vi "principal.vi"() -> ()   [LabVIEW 2020]
uses:
  <vilib>/Utility/file.llb/Read Delimited Spreadsheet (string).vi
  <vilib>/Utility/file.llb/Write Delimited Spreadsheet (string).vi
panel:
  in  "stop 2":bool
  in  "file path (dialog if empty) 2":path
  in  "stop":bool
  in  "file path (dialog if empty)":path
  out "appended path":path
  in  "CONTROL B":T1(tab)
  in  "Usuario 2":string
  in  "ingresar 2":bool
  in  "Contraseña 2":string
  out "String 4":string
  in  "volver 5":bool
  in  "Eliminar  2":bool
  in  "Agregar  2":bool
  in  "volver 6":bool
  in  "Agregar  10":bool
  in  "Contraseña nueva 2":string
  in  "Usuario nuevo 2":string
  out "String 3":string
  in  "volver 7":bool
  in  "Fila a eliminar 2":i32
  in  "Eliminar  4":bool
  out "all rows 2":string[][](array[string])
  in  "volver 10":bool
  out "Hora del sistema 2":string
  in  "volver 8":bool
  out "Nombre del usuario 2":string
  in  "CONTROL A":T2(tab)
  in  "ingresar":bool
  in  "Contraseña":string
  in  "Usuario":string
  in  "Agregar  3":bool
  in  "volver":bool
  in  "Eliminar":bool
  in  "Contraseña nueva":string
  in  "Usuario nuevo":string
  in  "volver 3":bool
  in  "Agregar":bool
  out "String":string
  in  "volver 4":bool
  out "all rows":string[][](array[string])
  in  "Fila a eliminar":i32
  in  "Eliminar  3":bool
  in  "volver 9":bool
  out "Hora del sistema":string
  out "Nombre del usuario":string
  in  "volver 2":bool
  # "INGRESAR"
  # "ADMINISTRADOR"
  # "PRINCIPAL"
  # "INGRESAR"
  # "ADMINISTRADOR"
  # "PRINCIPAL"
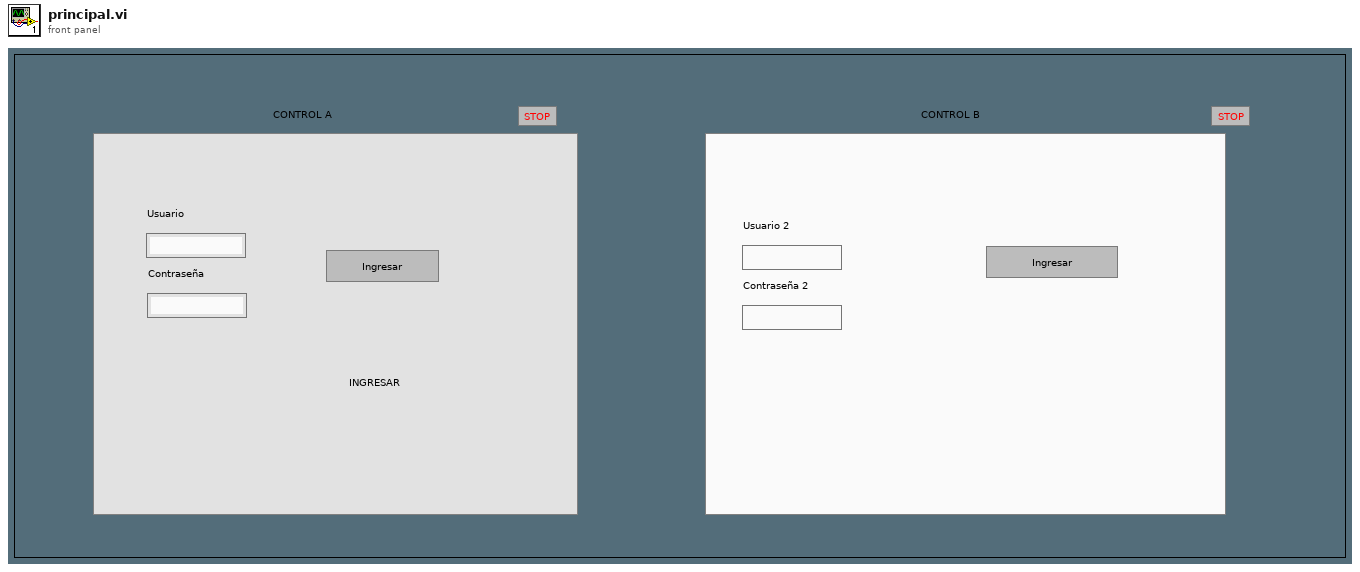
[diagram p1: front panel]
types:
  T1 = enum32{"INGRESAR", "ADMIN", "agregar ", "eliminar", "PRINCIPAL"}
  T2 = enum32{"INGRESAR", "ADMIN", "agregar", "eliminar", "PRINCIPAL"}
  T3 = enum16{"open", "replace", "create", "open or create", "replace or create", "replace or create with confirmation"}
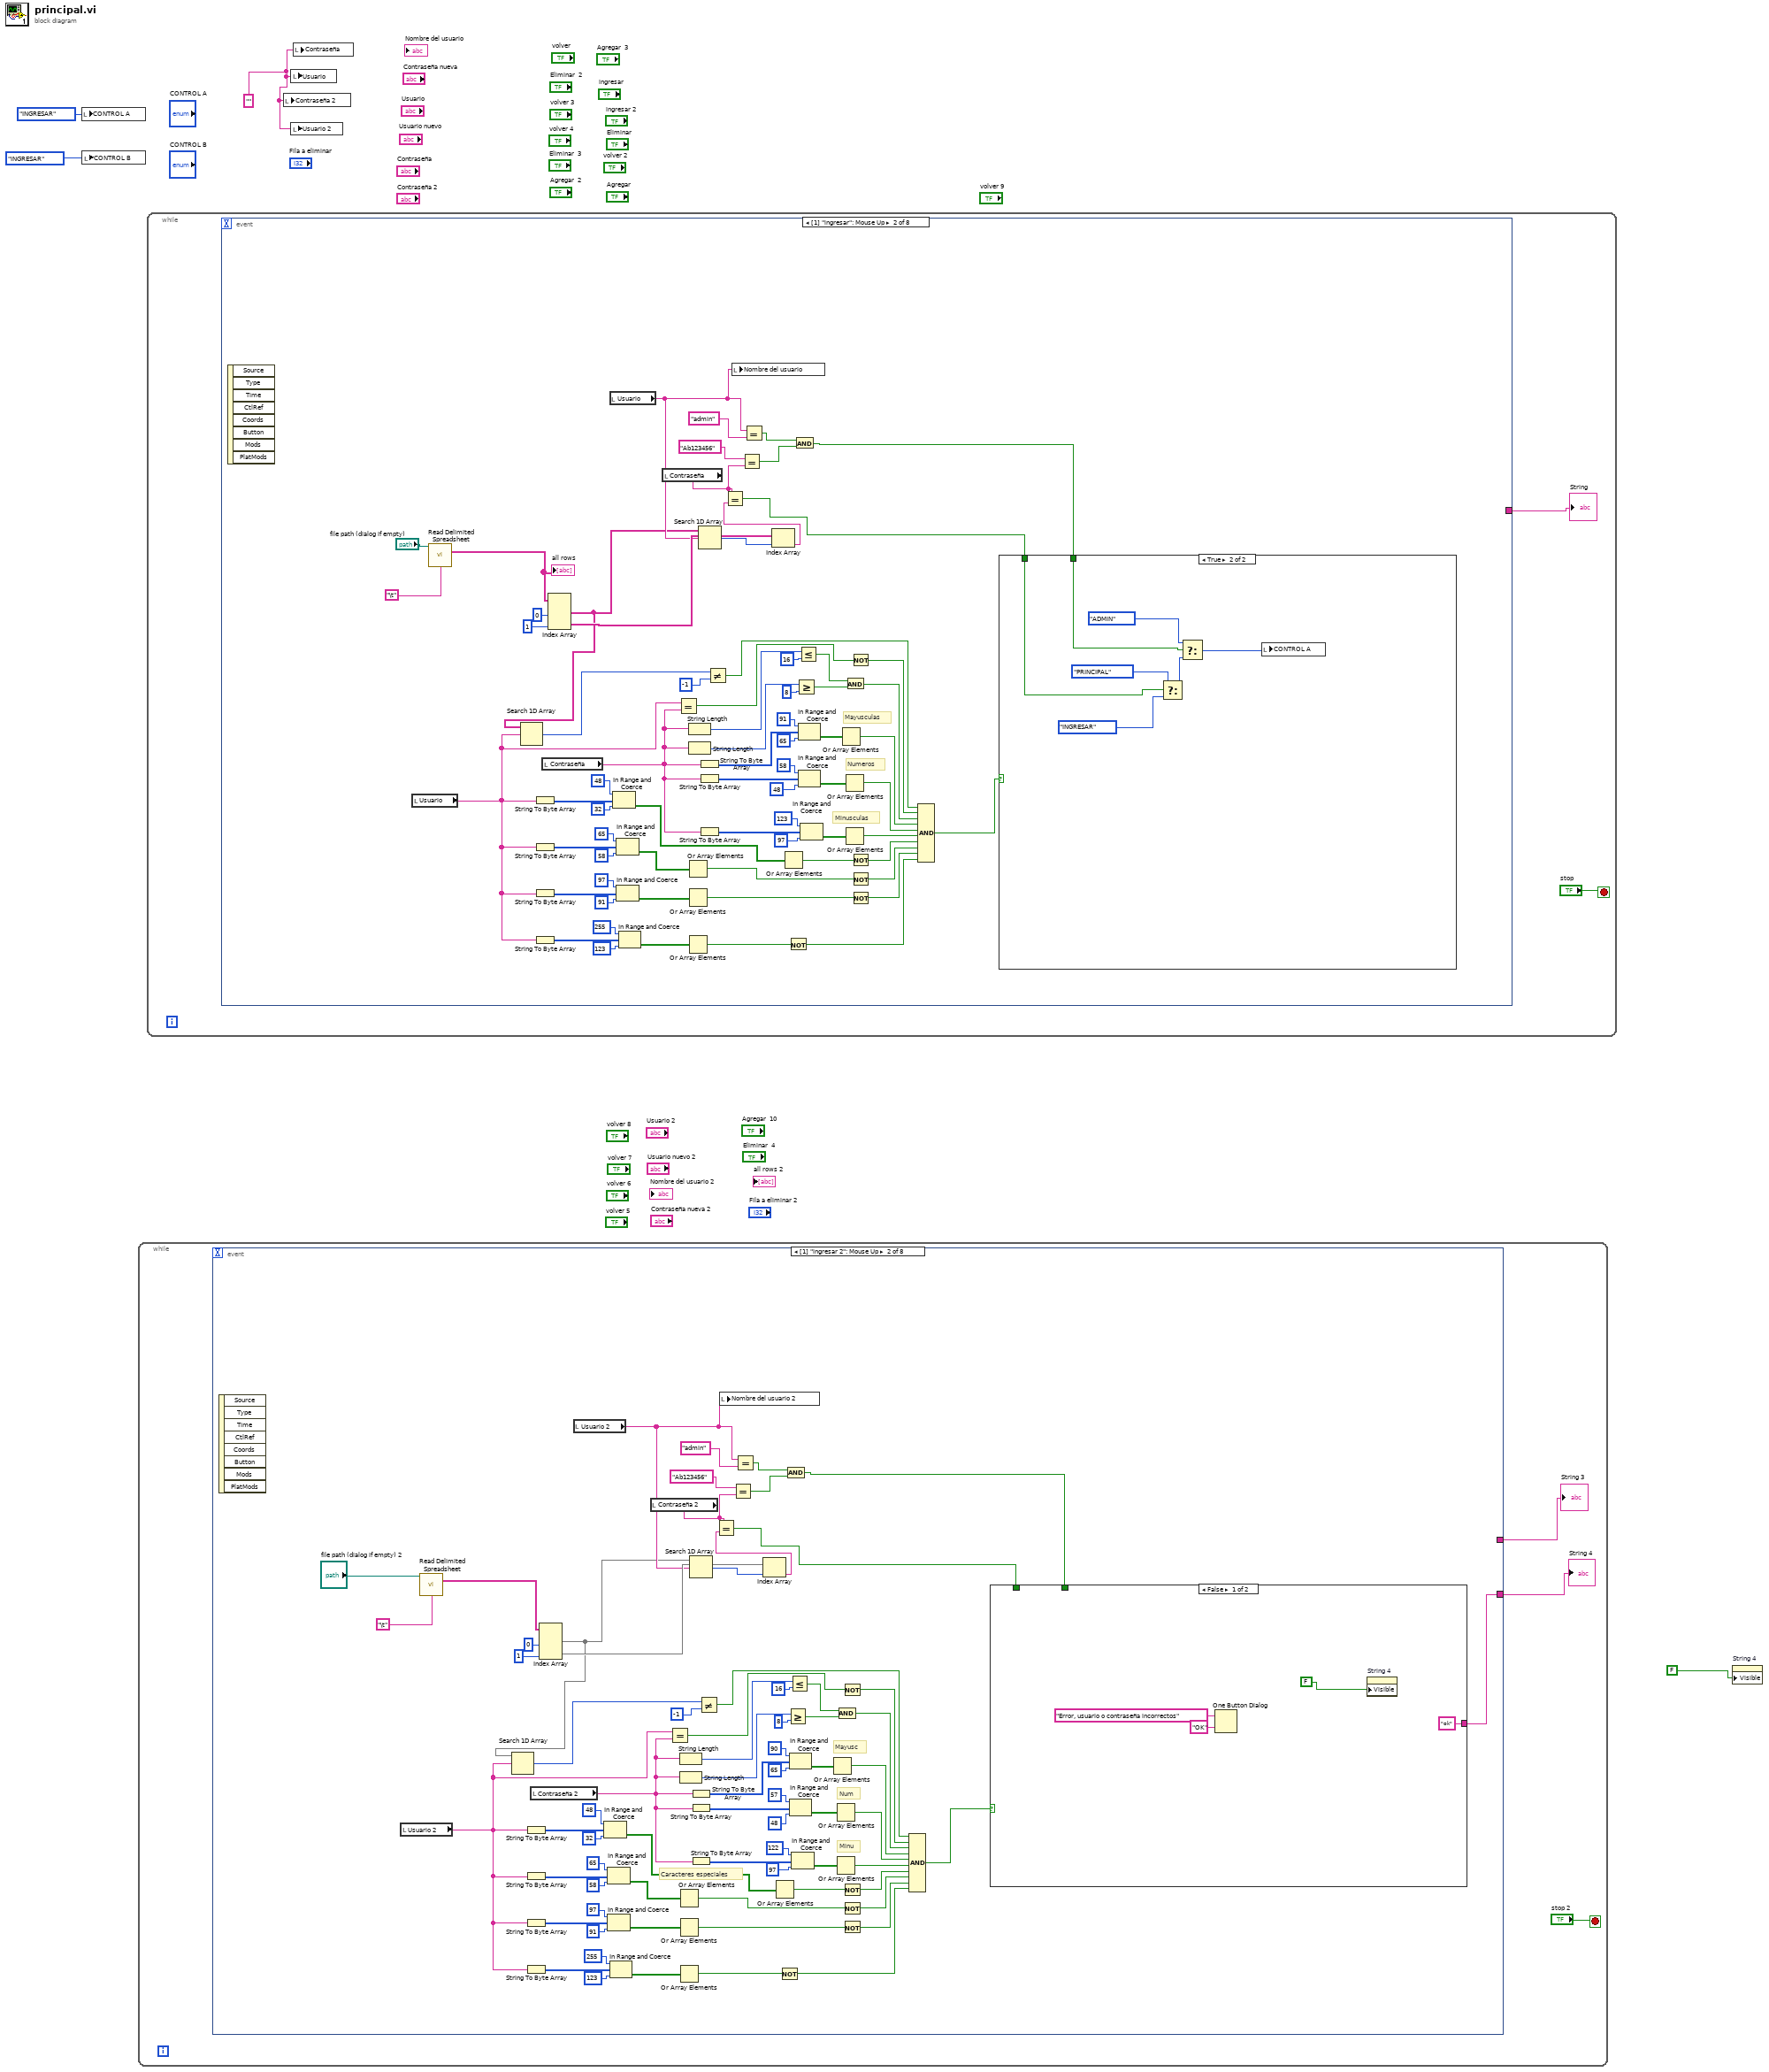
[diagram p0: block diagram]
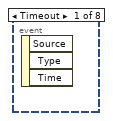
[diagram p2: hidden frame]
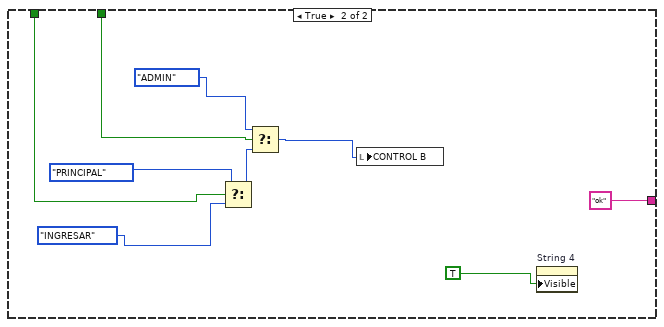
[diagram p3: hidden frame]
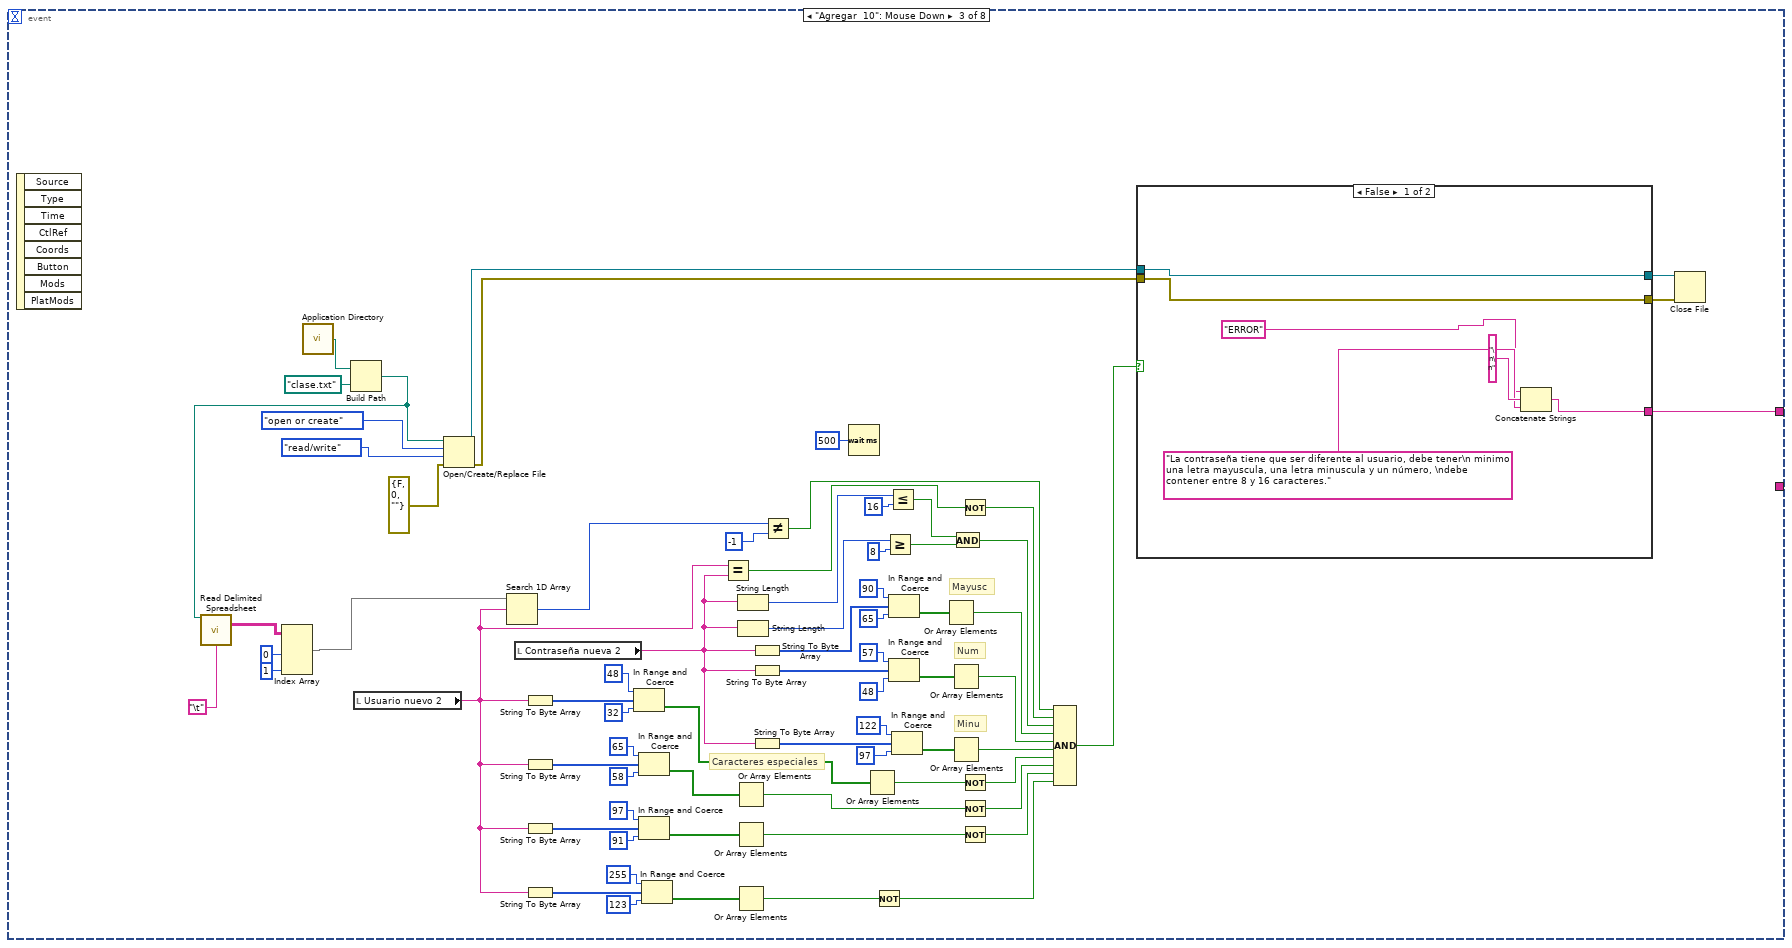
[diagram p4: hidden frame]
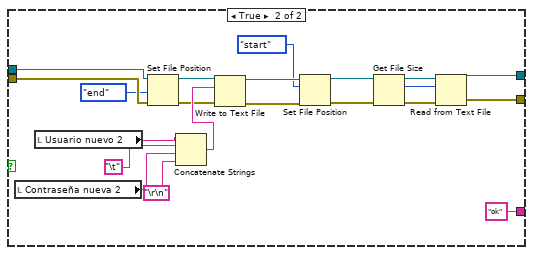
[diagram p5: hidden frame]
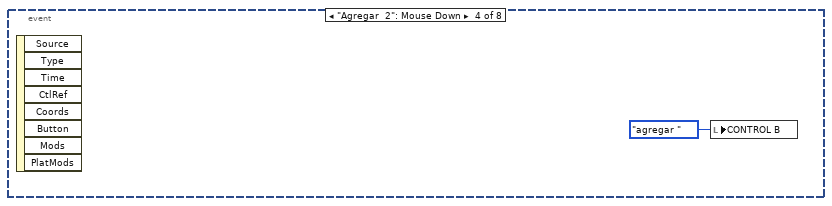
[diagram p6: hidden frame]
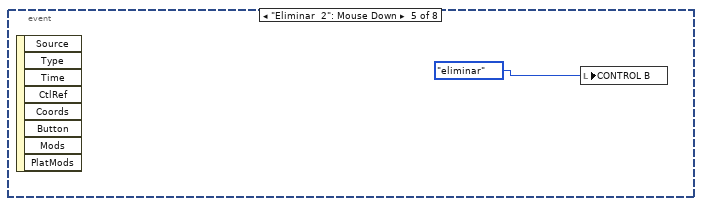
[diagram p7: hidden frame]
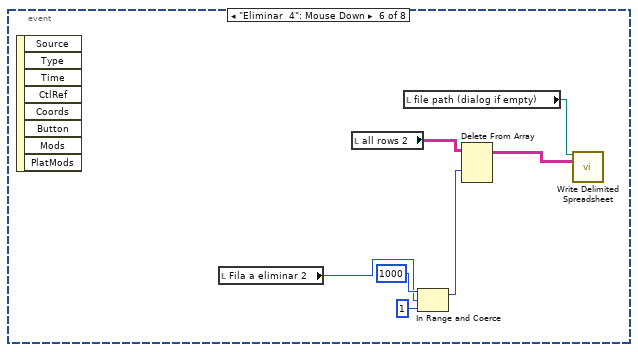
[diagram p8: hidden frame]
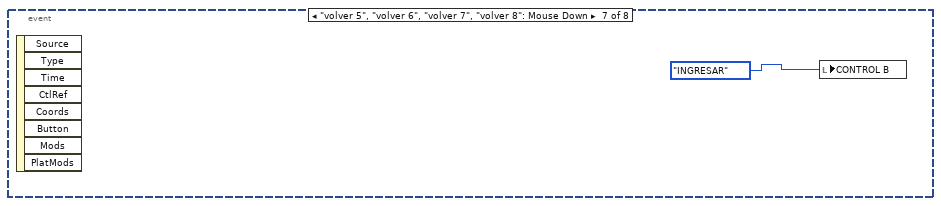
[diagram p9: hidden frame]
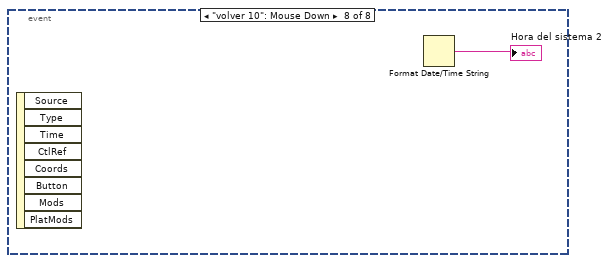
[diagram p10: hidden frame]
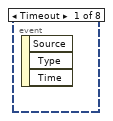
[diagram p11: hidden frame]
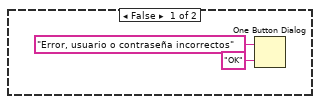
[diagram p12: hidden frame]
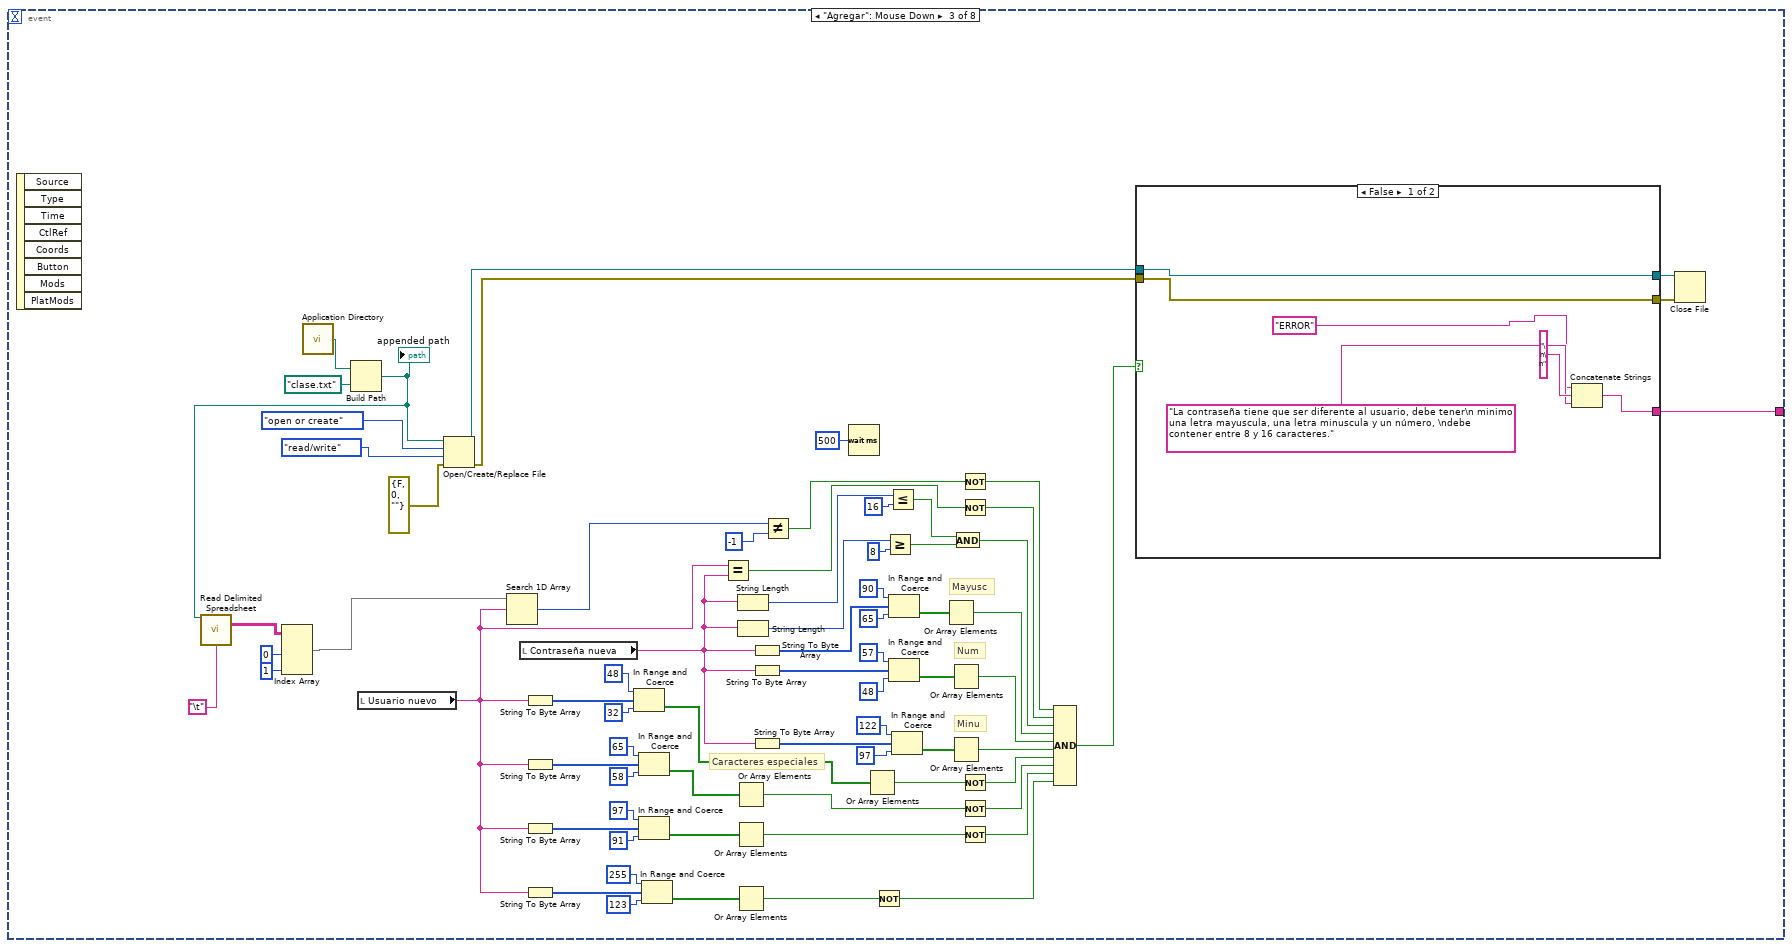
[diagram p13: hidden frame]
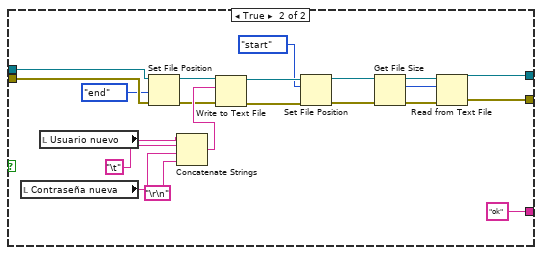
[diagram p14: hidden frame]
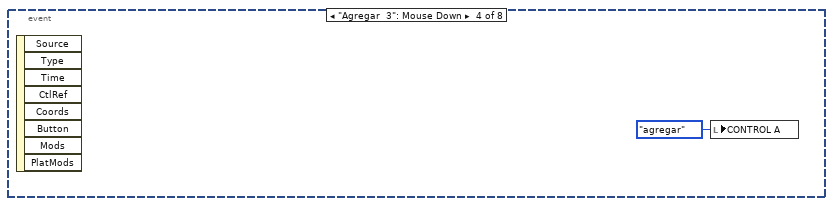
[diagram p15: hidden frame]
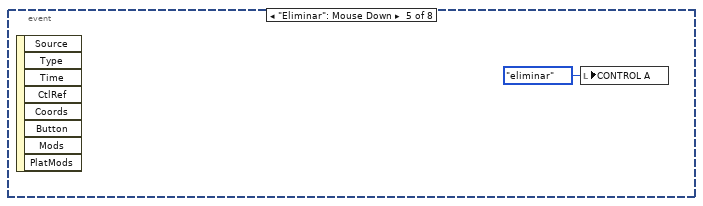
[diagram p16: hidden frame]
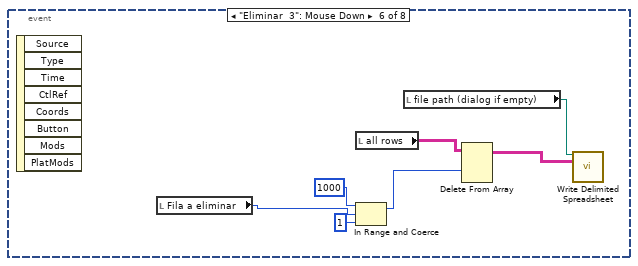
[diagram p17: hidden frame]
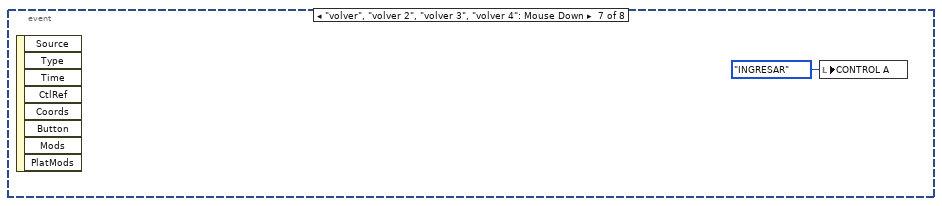
[diagram p18: hidden frame]
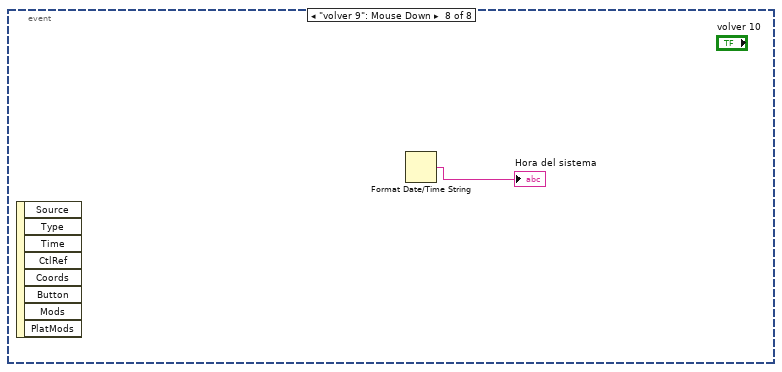
[diagram p19: hidden frame]
diagram:
  w2 = "" ("Usuario")
  n1 = local write "CONTROL A"(T2."INGRESAR" ("Tab Control")) -> ()
  n2 = local write "CONTROL B"(T1."INGRESAR" ("Tab Control 2")) -> ()
  n3 = while {
    stop <- "stop 2" stop-if-true
    n4 = event shown="[1] \"ingresar 2\": Mouse Up" {
      selector: _ -> [_ _ _ _ _ _ _ _]
      dyn-events: _ -> [_ _ _ _ _ _ _ _]
      timeout: _ -> [_ _ _ _ _ _ _ _]
      tunnel: [_ _ w94 _ _ _ _ _] -> w6
      tunnel: [_ w11 _ _ _ _ _ _] -> w5
      event Timeout {
        n5 = event-data() -> ()  [unwired: 1 in, 3 out]
      }
      event "ingresar 2": Mouse Up {
        # "Caracteres especiales"
        # "Minu"
        # "Num"
        # "Mayusc"
        n6 = event-data() -> ()  [unwired: 1 in, 8 out]
        n7 = local read "Usuario 2"() -> (w14:string)
        n8 = call-poly <vilib>:"Read Delimited Spreadsheet.vi"("file path (dialog if empty)"="file path (dialog if empty) 2", "delimiter (\\t)"="\t") -> ("all rows"=w74:string[][])  [unwired: 8 in, 5 out]
        n9 = String To Byte Array(string=w14) -> (unsigned byte array=w38:u8[])
        n10 = String To Byte Array(string=w14) -> (unsigned byte array=w33:u8[])
        n11 = String To Byte Array(string=w14) -> (unsigned byte array=w32:u8[])
        n12 = String To Byte Array(string=w14) -> (unsigned byte array=w23:u8[])
        n13 = local read "Contraseña 2"() -> (w41:string)
        n14 = Index Array(array=w74, index (col) #1=0 ("disabled index (col)"), index (col) #2=1 ("index (col)")) -> (element #1=w13:string[], element #2=w72:string[])  [unwired: 2 in]
        n15 = Search 1D Array(1D array=w13, element=w14) -> (index of element=w40:i32)  [unwired: 1 in]
        n16 = local read "Usuario 2"() -> (w66:string)
        n17 = In Range and Coerce(upper limit=u8 48, x=w38, lower limit=u8 32) -> (In Range?=w29:bool[])  [unwired: 1 out]
        n18 = In Range and Coerce(upper limit=u8 65, x=w33, lower limit=u8 58) -> (In Range?=w28:bool[])  [unwired: 1 out]
        n19 = In Range and Coerce(upper limit=u8 97, x=w32, lower limit=u8 91) -> (In Range?=w27:bool[])  [unwired: 1 out]
        n20 = In Range and Coerce(upper limit=u8 255, x=w23, lower limit=u8 123) -> (In Range?=w26:bool[])  [unwired: 1 out]
        n21 = local read "Contraseña 2"() -> (w68:string)
        n22 = Equal?(x=w14, y=w41) -> (x = y?=w43:bool)
        n23 = Or Array Elements(Boolean array=w28) -> (logical OR=w21:bool)
        n24 = Or Array Elements(Boolean array=w27) -> (logical OR=w20:bool)
        n25 = Or Array Elements(Boolean array=w26) -> (logical OR=w19:bool)
        n26 = String Length(string=w41) -> (length=w65:i32)
        n27 = String Length(string=w41) -> (length=w63:i32)
        n28 = Search 1D Array(1D array=w13, element=w66) -> (index of element=w71:i32)  [unwired: 1 in]
        n29 = String To Byte Array(string=w41) -> (unsigned byte array=w51:u8[])
        n30 = String To Byte Array(string=w41) -> (unsigned byte array=w52:u8[])
        n31 = String To Byte Array(string=w41) -> (unsigned byte array=w59:u8[])
        n32 = Not Equal?(x=w40, y=-1) -> (x != y?=w8:bool)
        n33 = local write "Nombre del usuario 2"(w66) -> ()
        n34 = Equal?(x="Ab123456", y=w68) -> (x = y?=w69:bool)
        n35 = Equal?(x=w66, y="admin") -> (x = y?=w78:bool)
        n36 = Index Array(array=w72, index=w71) -> (element=w70:string)
        n37 = Equal?(x=w68, y=w70) -> (x = y?=w10:bool)
        n38 = Or Array Elements(Boolean array=w29) -> (logical OR=w22:bool)
        n39 = Not(x=w19) -> (.not. x?=w15:bool)
        n40 = And(x=w78, y=w69) -> (x .and. y?=w9:bool)
        n41 = Greater Or Equal?(x=w63, y=8) -> (x >= y?=w60:bool)
        n42 = Less Or Equal?(x=w65, y=16) -> (x <= y?=w61:bool)
        n43 = In Range and Coerce(upper limit=u8 90, x=w51, lower limit=u8 65) -> (In Range?=w48:bool[])  [unwired: 1 out]
        n44 = In Range and Coerce(upper limit=u8 57, x=w52, lower limit=u8 48) -> (In Range?=w55:bool[])  [unwired: 1 out]
        n45 = In Range and Coerce(upper limit=u8 122, x=w59, lower limit=u8 97) -> (In Range?=w56:bool[])  [unwired: 1 out]
        n46 = Or Array Elements(Boolean array=w48) -> (logical OR=w46:bool)
        n47 = Or Array Elements(Boolean array=w55) -> (logical OR=w45:bool)
        n48 = Or Array Elements(Boolean array=w56) -> (logical OR=w44:bool)
        n49 = And(x=w61, y=w60) -> (x .and. y?=w47:bool)
        n50 = Not(x=w43) -> (.not. x?=w42:bool)
        n51 = Not(x=w22) -> (.not. x?=w18:bool)
        n52 = Not(x=w21) -> (.not. x?=w17:bool)
        n53 = Not(x=w20) -> (.not. x?=w16:bool)
        n54 = Compound Arithmetic op=AND(w8, w42, w47, w46, w45, w44, w18, w17, w16, w15) -> (w12:bool)
        n55 = case shown="False" w12 {
          tunnel: w9 -> [_ w89]
          tunnel: ["ok" "ok"] -> w11
          tunnel: w10 -> [_ w90]
          frame False {
            n56 = One Button Dialog(message="Error, usuario o contraseña incorrectos", button name ("OK")="OK") -> ()  [unwired: 1 out]
            n57 = property on="String 4" class="Str"("Visible"=FALSE) -> ()  [unwired: 2 in, 2 out]
          }
          frame True {
            n58 = Select(t=T1."PRINCIPAL" ("Tab Control 2"), s=w90, f=T1."INGRESAR" ("Tab Control 2")) -> (s? t:f=w92:T1)
            n59 = Select(t=T1."ADMIN" ("Tab Control 2"), s=w89, f=w92) -> (s? t:f=w88:T1)
            n60 = local write "CONTROL B"(w88) -> ()
            n61 = property on="String 4" class="Str"("Visible"=TRUE) -> ()  [unwired: 2 in, 2 out]
          }
        }
      }
      event "Agregar  10": Mouse Down {
        # "Caracteres especiales"
        # "Minu"
        # "Num"
        # "Mayusc"
        n62 = event-data() -> ()  [unwired: 1 in, 8 out]
        n63 = call <vilib>:"Application Directory.vi"() -> ("Application Directory"=w163:path)
        n64 = Build Path(base path=w163, name or relative path=path "clase.txt") -> (appended path=w105:path)
        n65 = call-poly <vilib>:"Read Delimited Spreadsheet.vi"("file path (dialog if empty)"=w105, "delimiter (\\t)"="\t") -> ("all rows"=w104:string[][])  [unwired: 8 in, 5 out]
        n66 = Index Array(array=w104, index (col) #1=0 ("disabled index (col)"), index (col) #2=1 ("index (col)")) -> (element #1=w100:string[])  [unwired: 2 in, 1 out]
        n67 = local read "Usuario nuevo 2"() -> (w114:string)
        n68 = Open/Create/Replace File(file path (use dialog)=w105, error in=errorcluster {"status"=FALSE, "code"=0, "source"=""}, operation (0:open)=T3."open or create", access (0:read/write)=enum16{"read/write", "read-only", "write-only"}."read/write") -> (refnum out=w97:refnum<file>, error out=w98:errorcluster)  [unwired: 2 in, 1 out]
        n69 = Search 1D Array(1D array=w100, element=w114) -> (index of element=w132:i32)  [unwired: 1 in]
        n70 = local read "Contraseña nueva 2"() -> (w133:string)
        n71 = String To Byte Array(string=w114) -> (unsigned byte array=w130:u8[])
        n72 = String To Byte Array(string=w114) -> (unsigned byte array=w125:u8[])
        n73 = String To Byte Array(string=w114) -> (unsigned byte array=w124:u8[])
        n74 = String To Byte Array(string=w114) -> (unsigned byte array=w115:u8[])
        n75 = In Range and Coerce(upper limit=u8 48, x=w130, lower limit=u8 32) -> (In Range?=w121:bool[])  [unwired: 1 out]
        n76 = In Range and Coerce(upper limit=u8 65, x=w125, lower limit=u8 58) -> (In Range?=w120:bool[])  [unwired: 1 out]
        n77 = In Range and Coerce(upper limit=u8 97, x=w124, lower limit=u8 91) -> (In Range?=w119:bool[])  [unwired: 1 out]
        n78 = In Range and Coerce(upper limit=u8 255, x=w115, lower limit=u8 123) -> (In Range?=w118:bool[])  [unwired: 1 out]
        n79 = Equal?(x=w114, y=w133) -> (x = y?=w135:bool)
        n80 = Or Array Elements(Boolean array=w120) -> (logical OR=w112:bool)
        n81 = Or Array Elements(Boolean array=w119) -> (logical OR=w111:bool)
        n82 = Or Array Elements(Boolean array=w118) -> (logical OR=w110:bool)
        n83 = String Length(string=w133) -> (length=w157:i32)
        n84 = String Length(string=w133) -> (length=w155:i32)
        n85 = String To Byte Array(string=w133) -> (unsigned byte array=w143:u8[])
        n86 = String To Byte Array(string=w133) -> (unsigned byte array=w144:u8[])
        n87 = String To Byte Array(string=w133) -> (unsigned byte array=w151:u8[])
        n88 = Not Equal?(x=w132, y=-1) -> (x != y?=w93:bool)
        n89 = Wait (ms)(milliseconds to wait=u32 500) -> ()  [unwired: 1 out]
        n90 = Or Array Elements(Boolean array=w121) -> (logical OR=w113:bool)
        n91 = Not(x=w110) -> (.not. x?=w106:bool)
        n92 = Greater Or Equal?(x=w155, y=8) -> (x >= y?=w152:bool)
        n93 = Less Or Equal?(x=w157, y=16) -> (x <= y?=w153:bool)
        n94 = In Range and Coerce(upper limit=u8 90, x=w143, lower limit=u8 65) -> (In Range?=w140:bool[])  [unwired: 1 out]
        n95 = In Range and Coerce(upper limit=u8 57, x=w144, lower limit=u8 48) -> (In Range?=w147:bool[])  [unwired: 1 out]
        n96 = In Range and Coerce(upper limit=u8 122, x=w151, lower limit=u8 97) -> (In Range?=w148:bool[])  [unwired: 1 out]
        n97 = Or Array Elements(Boolean array=w140) -> (logical OR=w138:bool)
        n98 = Or Array Elements(Boolean array=w147) -> (logical OR=w137:bool)
        n99 = Or Array Elements(Boolean array=w148) -> (logical OR=w136:bool)
        n100 = And(x=w153, y=w152) -> (x .and. y?=w139:bool)
        n101 = Not(x=w135) -> (.not. x?=w134:bool)
        n102 = Not(x=w113) -> (.not. x?=w109:bool)
        n103 = Not(x=w112) -> (.not. x?=w108:bool)
        n104 = Not(x=w111) -> (.not. x?=w107:bool)
        n105 = Compound Arithmetic op=AND(w93, w134, w139, w138, w137, w136, w109, w108, w107, w106) -> (w99:bool)
        n106 = case shown="False" w99 {
          tunnel: w98 -> [w168 w175]
          tunnel: w97 -> [w169 w173]
          tunnel: [w168 w172] -> w96
          tunnel: [w169 w171] -> w95
          tunnel: [w164 "ok"] -> w94
          frame False {
            n107 = Concatenate Strings("ERROR", "\n\n" ("string"), "La contraseña tiene que ser diferente al usuario, debe tener\n minimo una letra mayuscula, una letra minuscula y un número, \ndebe contener entre 8 y 16 caracteres.") -> (w164:string)
          }
          frame True {
            n108 = local read "Contraseña nueva 2"() -> (w190:string)
            n109 = local read "Usuario nuevo 2"() -> (w189:string)
            n110 = Set File Position(refnum=w173, from (0:start)=enum16{"start", "end", "current"}."end", error in=w175) -> (refnum out=w179:refnum<file>, error out=w182:errorcluster)  [unwired: 1 in]
            n111 = Concatenate Strings(w189, "\t", w190, "\r\n") -> (w188:string)
            n112 = Write to Text File(file (use dialog)=w179, text=w188, error in=w182) -> (refnum out=w180:refnum<file>, error out=w183:errorcluster)  [unwired: 1 in, 1 out]
            n113 = Set File Position(offset (in bytes) (0)=enum16{"start", "end", "current"}."start" ("from (0:start)"), refnum=w180, error in=w183) -> (refnum out=w181:refnum<file>, error out=w184:errorcluster)  [unwired: 1 in]
            n114 = Get File Size(file=w181, error in=w184) -> (refnum out=w185:refnum<file>, size (in bytes)=w187:i64, 0:w186:errorcluster)
            n115 = Read from Text File(file (use dialog)=w185, count=w187, error in=w186) -> (refnum out=w171:refnum<file>, error out=w172:errorcluster)  [unwired: 1 in, 2 out]
          }
        }
        n116 = Close File(refnum=w95, error in=w96) -> ()  [unwired: 2 out]
      }
      event "Agregar  2": Mouse Down {
        n117 = event-data() -> ()  [unwired: 1 in, 8 out]
        n118 = local write "CONTROL B"(T1."agregar " ("Tab Control 2")) -> ()
      }
      event "Eliminar  2": Mouse Down {
        n119 = event-data() -> ()  [unwired: 1 in, 8 out]
        n120 = local write "CONTROL B"(T1."eliminar" ("Tab Control 2")) -> ()
      }
      event "Eliminar  4": Mouse Down {
        n121 = event-data() -> ()  [unwired: 1 in, 8 out]
        n122 = local read "Fila a eliminar 2"() -> (w194:i32)
        n123 = local read "all rows 2"() -> (w198:string[][])
        n124 = local read "file path (dialog if empty)"() -> (w199:path)
        n125 = In Range and Coerce(upper limit=1000, x=w194, lower limit=1) -> (coerced(x)=w193:i32)  [unwired: 1 out]
        n126 = Delete From Array(array=w198, index (row)=w193) -> (array with subset deleted=w197:string[][])  [unwired: 2 in, 1 out]
        n127 = call-poly <vilib>:"Write Delimited Spreadsheet.vi"("file path (dialog if empty)"=w199, "2D data"=w197) -> ()  [unwired: 12 in, 2 out]
      }
      event "volver 5", "volver 6", "volver 7", "volver 8": Mouse Down {
        n128 = event-data() -> ()  [unwired: 1 in, 8 out]
        n129 = local write "CONTROL B"(T1."INGRESAR" ("Tab Control 2")) -> ()
      }
      event "volver 10": Mouse Down {
        n130 = event-data() -> ()  [unwired: 1 in, 8 out]
        n131 = Format Date/Time String() -> (date/time string=→"Hora del sistema 2":string)  [unwired: 3 in]
      }
    }
    "String 3" <- w6
    "String 4" <- w5
  }
  n132 = while {
    stop <- "stop" stop-if-true
    n133 = event shown="[1] \"ingresar\": Mouse Up" {
      selector: _ -> [_ _ _ _ _ _ _ _]
      dyn-events: _ -> [_ _ _ _ _ _ _ _]
      timeout: _ -> [_ _ _ _ _ _ _ _]
      tunnel: [_ _ w284 _ _ _ _ _] -> w202
      event Timeout {
        n134 = event-data() -> ()  [unwired: 1 in, 3 out]
      }
      event "ingresar": Mouse Up {
        # "Minusculas"
        # "Numeros"
        # "Mayusculas"
        n135 = event-data() -> ()  [unwired: 1 in, 8 out]
        n136 = local read "Usuario"() -> (w209:string)
        n137 = call-poly <vilib>:"Read Delimited Spreadsheet.vi"("file path (dialog if empty)"="file path (dialog if empty)", "delimiter (\\t)"="\t") -> ("all rows"=w269:string[][])  [unwired: 8 in, 5 out]
        "all rows" <- w269
        n138 = String To Byte Array(string=w209) -> (unsigned byte array=w233:u8[])
        n139 = String To Byte Array(string=w209) -> (unsigned byte array=w228:u8[])
        n140 = String To Byte Array(string=w209) -> (unsigned byte array=w227:u8[])
        n141 = String To Byte Array(string=w209) -> (unsigned byte array=w218:u8[])
        n142 = local read "Contraseña"() -> (w236:string)
        n143 = Index Array(array=w269, index (col) #1=0 ("disabled index (col)"), index (col) #2=1 ("index (col)")) -> (element #1=w208:string[], element #2=w267:string[])  [unwired: 2 in]
        n144 = Search 1D Array(1D array=w208, element=w209) -> (index of element=w235:i32)  [unwired: 1 in]
        n145 = local read "Usuario"() -> (w261:string)
        n146 = In Range and Coerce(upper limit=u8 48, x=w233, lower limit=u8 32) -> (In Range?=w224:bool[])  [unwired: 1 out]
        n147 = In Range and Coerce(upper limit=u8 65, x=w228, lower limit=u8 58) -> (In Range?=w223:bool[])  [unwired: 1 out]
        n148 = In Range and Coerce(upper limit=u8 97, x=w227, lower limit=u8 91) -> (In Range?=w222:bool[])  [unwired: 1 out]
        n149 = In Range and Coerce(upper limit=u8 255, x=w218, lower limit=u8 123) -> (In Range?=w221:bool[])  [unwired: 1 out]
        n150 = local read "Contraseña"() -> (w263:string)
        n151 = Equal?(x=w209, y=w236) -> (x = y?=w238:bool)
        n152 = Or Array Elements(Boolean array=w223) -> (logical OR=w216:bool)
        n153 = Or Array Elements(Boolean array=w222) -> (logical OR=w215:bool)
        n154 = Or Array Elements(Boolean array=w221) -> (logical OR=w214:bool)
        n155 = String Length(string=w236) -> (length=w260:i32)
        n156 = String Length(string=w236) -> (length=w258:i32)
        n157 = Search 1D Array(1D array=w208, element=w261) -> (index of element=w266:i32)  [unwired: 1 in]
        n158 = String To Byte Array(string=w236) -> (unsigned byte array=w246:u8[])
        n159 = String To Byte Array(string=w236) -> (unsigned byte array=w247:u8[])
        n160 = String To Byte Array(string=w236) -> (unsigned byte array=w254:u8[])
        n161 = Not Equal?(x=w235, y=-1) -> (x != y?=w204:bool)
        n162 = local write "Nombre del usuario"(w261) -> ()
        n163 = Equal?(x="Ab123456", y=w263) -> (x = y?=w264:bool)
        n164 = Equal?(x=w261, y="admin") -> (x = y?=w273:bool)
        n165 = Index Array(array=w267, index=w266) -> (element=w265:string)
        n166 = Equal?(x=w263, y=w265) -> (x = y?=w206:bool)
        n167 = Or Array Elements(Boolean array=w224) -> (logical OR=w217:bool)
        n168 = Not(x=w214) -> (.not. x?=w210:bool)
        n169 = And(x=w273, y=w264) -> (x .and. y?=w205:bool)
        n170 = Greater Or Equal?(x=w258, y=8) -> (x >= y?=w255:bool)
        n171 = Less Or Equal?(x=w260, y=16) -> (x <= y?=w256:bool)
        n172 = In Range and Coerce(upper limit=u8 91, x=w246, lower limit=u8 65) -> (In Range?=w243:bool[])  [unwired: 1 out]
        n173 = In Range and Coerce(upper limit=u8 58, x=w247, lower limit=u8 48) -> (In Range?=w250:bool[])  [unwired: 1 out]
        n174 = In Range and Coerce(upper limit=u8 123, x=w254, lower limit=u8 97) -> (In Range?=w251:bool[])  [unwired: 1 out]
        n175 = Or Array Elements(Boolean array=w243) -> (logical OR=w241:bool)
        n176 = Or Array Elements(Boolean array=w250) -> (logical OR=w240:bool)
        n177 = Or Array Elements(Boolean array=w251) -> (logical OR=w239:bool)
        n178 = And(x=w256, y=w255) -> (x .and. y?=w242:bool)
        n179 = Not(x=w238) -> (.not. x?=w237:bool)
        n180 = Not(x=w217) -> (.not. x?=w213:bool)
        n181 = Not(x=w216) -> (.not. x?=w212:bool)
        n182 = Not(x=w215) -> (.not. x?=w211:bool)
        n183 = Compound Arithmetic op=AND(w204, w237, w242, w241, w240, w239, w213, w212, w211, w210) -> (w207:bool)
        n184 = case shown="True" w207 {
          tunnel: w205 -> [_ w277]
          tunnel: w206 -> [_ w278]
          frame False {
            n185 = One Button Dialog(message="Error, usuario o contraseña incorrectos", button name ("OK")="OK") -> ()  [unwired: 1 out]
          }
          frame True {
            n186 = Select(t=T2."PRINCIPAL" ("Tab Control"), s=w278, f=T2."INGRESAR" ("Tab Control")) -> (s? t:f=w282:T2)
            n187 = Select(t=T2."ADMIN" ("Tab Control"), s=w277, f=w282) -> (s? t:f=w283:T2)
            n188 = local write "CONTROL A"(w283) -> ()
          }
        }
      }
      event "Agregar": Mouse Down {
        # "Caracteres especiales"
        # "Minu"
        # "Num"
        # "Mayusc"
        n189 = event-data() -> ()  [unwired: 1 in, 8 out]
        n190 = call <vilib>:"Application Directory.vi"() -> ("Application Directory"=w355:path)
        n191 = Build Path(base path=w355, name or relative path=path "clase.txt") -> (appended path=w295:path)
        "appended path" <- w295
        n192 = call-poly <vilib>:"Read Delimited Spreadsheet.vi"("file path (dialog if empty)"=w295, "delimiter (\\t)"="\t") -> ("all rows"=w294:string[][])  [unwired: 8 in, 5 out]
        n193 = Index Array(array=w294, index (col) #1=0 ("disabled index (col)"), index (col) #2=1 ("index (col)")) -> (element #1=w290:string[])  [unwired: 2 in, 1 out]
        n194 = local read "Usuario nuevo"() -> (w304:string)
        n195 = Open/Create/Replace File(file path (use dialog)=w295, error in=errorcluster {"status"=FALSE, "code"=0, "source"=""}, operation (0:open)=T3."open or create", access (0:read/write)=enum16{"read/write", "read-only", "write-only"}."read/write") -> (refnum out=w287:refnum<file>, error out=w288:errorcluster)  [unwired: 2 in, 1 out]
        n196 = Search 1D Array(1D array=w290, element=w304) -> (index of element=w324:i32)  [unwired: 1 in]
        n197 = local read "Contraseña nueva"() -> (w325:string)
        n198 = String To Byte Array(string=w304) -> (unsigned byte array=w320:u8[])
        n199 = String To Byte Array(string=w304) -> (unsigned byte array=w315:u8[])
        n200 = String To Byte Array(string=w304) -> (unsigned byte array=w314:u8[])
        n201 = String To Byte Array(string=w304) -> (unsigned byte array=w305:u8[])
        n202 = In Range and Coerce(upper limit=u8 48, x=w320, lower limit=u8 32) -> (In Range?=w311:bool[])  [unwired: 1 out]
        n203 = In Range and Coerce(upper limit=u8 65, x=w315, lower limit=u8 58) -> (In Range?=w310:bool[])  [unwired: 1 out]
        n204 = In Range and Coerce(upper limit=u8 97, x=w314, lower limit=u8 91) -> (In Range?=w309:bool[])  [unwired: 1 out]
        n205 = In Range and Coerce(upper limit=u8 255, x=w305, lower limit=u8 123) -> (In Range?=w308:bool[])  [unwired: 1 out]
        n206 = Equal?(x=w304, y=w325) -> (x = y?=w327:bool)
        n207 = Or Array Elements(Boolean array=w310) -> (logical OR=w302:bool)
        n208 = Or Array Elements(Boolean array=w309) -> (logical OR=w301:bool)
        n209 = Or Array Elements(Boolean array=w308) -> (logical OR=w300:bool)
        n210 = String Length(string=w325) -> (length=w349:i32)
        n211 = String Length(string=w325) -> (length=w347:i32)
        n212 = String To Byte Array(string=w325) -> (unsigned byte array=w335:u8[])
        n213 = String To Byte Array(string=w325) -> (unsigned byte array=w336:u8[])
        n214 = String To Byte Array(string=w325) -> (unsigned byte array=w343:u8[])
        n215 = Not Equal?(x=w324, y=-1) -> (x != y?=w322:bool)
        n216 = Wait (ms)(milliseconds to wait=u32 500) -> ()  [unwired: 1 out]
        n217 = Or Array Elements(Boolean array=w311) -> (logical OR=w303:bool)
        n218 = Not(x=w300) -> (.not. x?=w296:bool)
        n219 = Greater Or Equal?(x=w347, y=8) -> (x >= y?=w344:bool)
        n220 = Less Or Equal?(x=w349, y=16) -> (x <= y?=w345:bool)
        n221 = In Range and Coerce(upper limit=u8 90, x=w335, lower limit=u8 65) -> (In Range?=w332:bool[])  [unwired: 1 out]
        n222 = In Range and Coerce(upper limit=u8 57, x=w336, lower limit=u8 48) -> (In Range?=w339:bool[])  [unwired: 1 out]
        n223 = In Range and Coerce(upper limit=u8 122, x=w343, lower limit=u8 97) -> (In Range?=w340:bool[])  [unwired: 1 out]
        n224 = Or Array Elements(Boolean array=w332) -> (logical OR=w330:bool)
        n225 = Or Array Elements(Boolean array=w339) -> (logical OR=w329:bool)
        n226 = Or Array Elements(Boolean array=w340) -> (logical OR=w328:bool)
        n227 = And(x=w345, y=w344) -> (x .and. y?=w331:bool)
        n228 = Not(x=w322) -> (.not. x?=w321:bool)
        n229 = Not(x=w327) -> (.not. x?=w326:bool)
        n230 = Not(x=w303) -> (.not. x?=w299:bool)
        n231 = Not(x=w302) -> (.not. x?=w298:bool)
        n232 = Not(x=w301) -> (.not. x?=w297:bool)
        n233 = Compound Arithmetic op=AND(w321, w326, w331, w330, w329, w328, w299, w298, w297, w296) -> (w289:bool)
        n234 = case shown="False" w289 {
          tunnel: w288 -> [w357 w367]
          tunnel: w287 -> [w358 w365]
          tunnel: [w357 w364] -> w286
          tunnel: [w358 w363] -> w285
          tunnel: [w359 "ok"] -> w284
          frame False {
            n235 = Concatenate Strings("ERROR", "\n\n" ("string"), "La contraseña tiene que ser diferente al usuario, debe tener\n minimo una letra mayuscula, una letra minuscula y un número, \ndebe contener entre 8 y 16 caracteres.") -> (w359:string)
          }
          frame True {
            n236 = local read "Contraseña nueva"() -> (w382:string)
            n237 = local read "Usuario nuevo"() -> (w381:string)
            n238 = Set File Position(refnum=w365, from (0:start)=enum16{"start", "end", "current"}."end", error in=w367) -> (refnum out=w371:refnum<file>, error out=w374:errorcluster)  [unwired: 1 in]
            n239 = Concatenate Strings(w381, "\t", w382, "\r\n") -> (w380:string)
            n240 = Write to Text File(file (use dialog)=w371, text=w380, error in=w374) -> (refnum out=w372:refnum<file>, error out=w375:errorcluster)  [unwired: 1 in, 1 out]
            n241 = Set File Position(offset (in bytes) (0)=enum16{"start", "end", "current"}."start" ("from (0:start)"), refnum=w372, error in=w375) -> (refnum out=w373:refnum<file>, error out=w376:errorcluster)  [unwired: 1 in]
            n242 = Get File Size(file=w373, error in=w376) -> (refnum out=w377:refnum<file>, size (in bytes)=w379:i64, 0:w378:errorcluster)
            n243 = Read from Text File(file (use dialog)=w377, count=w379, error in=w378) -> (refnum out=w363:refnum<file>, error out=w364:errorcluster)  [unwired: 1 in, 2 out]
          }
        }
        n244 = Close File(refnum=w285, error in=w286) -> ()  [unwired: 2 out]
      }
      event "Agregar  3": Mouse Down {
        n245 = event-data() -> ()  [unwired: 1 in, 8 out]
        n246 = local write "CONTROL A"(T2."agregar" ("Tab Control")) -> ()
      }
      event "Eliminar": Mouse Down {
        n247 = event-data() -> ()  [unwired: 1 in, 8 out]
        n248 = local write "CONTROL A"(T2."eliminar" ("Tab Control")) -> ()
      }
      event "Eliminar  3": Mouse Down {
        n249 = event-data() -> ()  [unwired: 1 in, 8 out]
        n250 = local read "Fila a eliminar"() -> (w388:i32)
        n251 = local read "all rows"() -> (w390:string[][])
        n252 = In Range and Coerce(upper limit=1000, x=w388, lower limit=1) -> (coerced(x)=w385:i32)  [unwired: 1 out]
        n253 = local read "file path (dialog if empty)"() -> (w391:path)
        n254 = Delete From Array(array=w390, index (row)=w385) -> (array with subset deleted=w389:string[][])  [unwired: 2 in, 1 out]
        n255 = call-poly <vilib>:"Write Delimited Spreadsheet.vi"("file path (dialog if empty)"=w391, "2D data"=w389) -> ()  [unwired: 12 in, 2 out]
      }
      event "volver", "volver 2", "volver 3", "volver 4": Mouse Down {
        n256 = event-data() -> ()  [unwired: 1 in, 8 out]
        n257 = local write "CONTROL A"(T2."INGRESAR" ("Tab Control")) -> ()
      }
      event "volver 9": Mouse Down {
        n258 = event-data() -> ()  [unwired: 1 in, 8 out]
        n259 = Format Date/Time String() -> (date/time string=→"Hora del sistema":string)  [unwired: 3 in]
      }
    }
    "String" <- w202
  }
  n260 = local write "Contraseña 2"(w2) -> ()
  n261 = local write "Usuario"(w2) -> ()
  n262 = local write "Usuario 2"(w2) -> ()
  n263 = local write "Contraseña"(w2) -> ()
  n264 = property on="String 4" class="Str"("Visible"=FALSE) -> ()  [unwired: 2 in, 2 out]
